vi "labviewRT_sm_example_waveform.vi"() -> ()   [LabVIEW 2019]
uses:
  lib/labviewRT-EPICS/linuxSharedMemory.lvlib
  lib/labviewRT-EPICS/sm u64 write and increment.vi
  lib/labviewRT-EPICS/sm single array write and increment.vi
  lib/labviewRT-EPICS/sm u64 write array and increment.vi
  lib/labviewRT-EPICS/sm u16 write array and increment.vi
  lib/labviewRT-EPICS/sm i64 write array and increment.vi
  lib/labviewRT-EPICS/sm double array write and increment.vi
  lib/labviewRT-EPICS/sm u32 write array and increment.vi
  lib/labviewRT-EPICS/sm i32 write and increment.vi
  lib/labviewRT-EPICS/sm u32 write and increment.vi
  lib/labviewRT-EPICS/sm u16 write and increment.vi
  lib/labviewRT-EPICS/sm i8 write and increment.vi
  lib/labviewRT-EPICS/sm bool write and increment.vi
  lib/labviewRT-EPICS/sm u8 write and increment.vi
  lib/labviewRT-EPICS/sm double write and increment.vi
  lib/labviewRT-EPICS/sm i8 write array and increment.vi
  lib/labviewRT-EPICS/sm i64 read and increment.vi
  lib/labviewRT-EPICS/sm i32 write array and increment.vi
  lib/labviewRT-EPICS/sm i16 write array and increment.vi
  lib/labviewRT-EPICS/sm bool array write and increment.vi
  lib/labviewRT-EPICS/sm u8 read and increment.vi
  lib/labviewRT-EPICS/sm u16 read and increment.vi
  lib/labviewRT-EPICS/sm i16 read and increment.vi
  lib/labviewRT-EPICS/sm u64 read and increment.vi
  lib/labviewRT-EPICS/sm i8 read and increment.vi
  lib/labviewRT-EPICS/sm single read and increment.vi
  lib/labviewRT-EPICS/sm i32 read and increment.vi
  lib/labviewRT-EPICS/sm single write and increment.vi
  lib/labviewRT-EPICS/sm u32 read and increment.vi
  lib/labviewRT-EPICS/sm i64 write and increment.vi
  lib/labviewRT-EPICS/sm u8 write array and increment.vi
  lib/labviewRT-EPICS/sm i16 write and increment.vi
  lib/labviewRT-EPICS/sm double read and increment.vi
  lib/labviewRT-EPICS/sm bool read and increment.vi
panel:
  in  "Boolean in scalar":bool
  in  "U8 scalar":u8
  in  "U16 scalar":u16
  in  "U32 scalar":u32
  in  "U64 scalar":u64
  in  "I8 scalar":i8
  in  "I16 scalar":i16
  in  "I32 scalar":i32
  in  "I64 scalar":i64
  in  "Sgl scalar":sgl format="%#_64g"
  in  "Dbl scalar":dbl format="%#_64g"
  out "U8 scalar":u8
  out "U16 scalar":u16
  out "U32 scalar":u32
  out "U64 scalar":u64
  out "I8 scalar":i8
  out "I16 scalar":i16
  out "I32 scalar":i32
  out "I64 scalar":i64
  out "Sgl  scalar":sgl format="%#_64g"
  out "Dbl scalar":dbl format="%#_64g"
  out "Boolean scalar":bool
  in  "stop":bool
  out "error out":errorcluster
  in  "u64 scaler":u64
  in  "i32":i32[](array[numeric])=[0, 0, 0, 0, 0, 0, 0, 0, 0, 1]
  in  "i16":i16[](array[numeric])=[0, 0, 0, 1]
  in  "i8":i8[](array[numeric])=[0, 0, 0, 0, 0, 0, 0, 1]
  in  "bool":bool[](array[boolean])=[FALSE, FALSE, FALSE, FALSE, FALSE, TRUE]
  in  "u64":u64[](array[numeric])=[0, 0, 0, 0, 0, 0, 0, 0, 1]
  in  "u16":u16[](array[numeric])=[0, 0, 0, 0, 0, 0, 0, 0, 0, 0, 1]
  in  "i64":i64[](array[numeric])=[0, 0, 0, 0, 1]
  in  "u8":u8[](array[numeric])=[0, 0, 0, 0, 0, 0, 0, 0, 1]
  out "Bool out":bool
  in  "double":dbl[](array[numeric])=[0.0, 0.0, 0.0, 1.0]
  in  "Shared Memory Size (bytes)":u32=4096
  in  "u32":u32[](array[numeric])=[0, 0, 0, 0, 0, 0, 0, 0, 0, 0, 0, 0, 0, 0, 0, 0, 0, 0, 0, 0, 0, 0, 0, 0, 0, 0, 0, 0, 0, 0, 0, 0, 0, 0, 0, 0, 0, 0, 0, 0, 0, 0, 0, 0, 0, 0, 0, 0, 0, 0, 0, 0, 0, 0, 0, 0, 0, 0, 0, 0, 0, 0, 0, 0, 0, 0, 0, 0, 0, 0, 0, 0, 0, 0, 0, 0, 0, 0, 0, 0, 0, 0, 0, 0, 0, 0, 0, 0, 0, 0, 0, 0, 0, 0, 0, 0, 0, 0, 0, 0, 0, 0, 0, 0, 0, 0, 0, 0, 0, 0, 0, 0, 1]
  in  "single":sgl[](array[numeric])=[0.0, 0.0, 0.0, 0.0, 1.0]
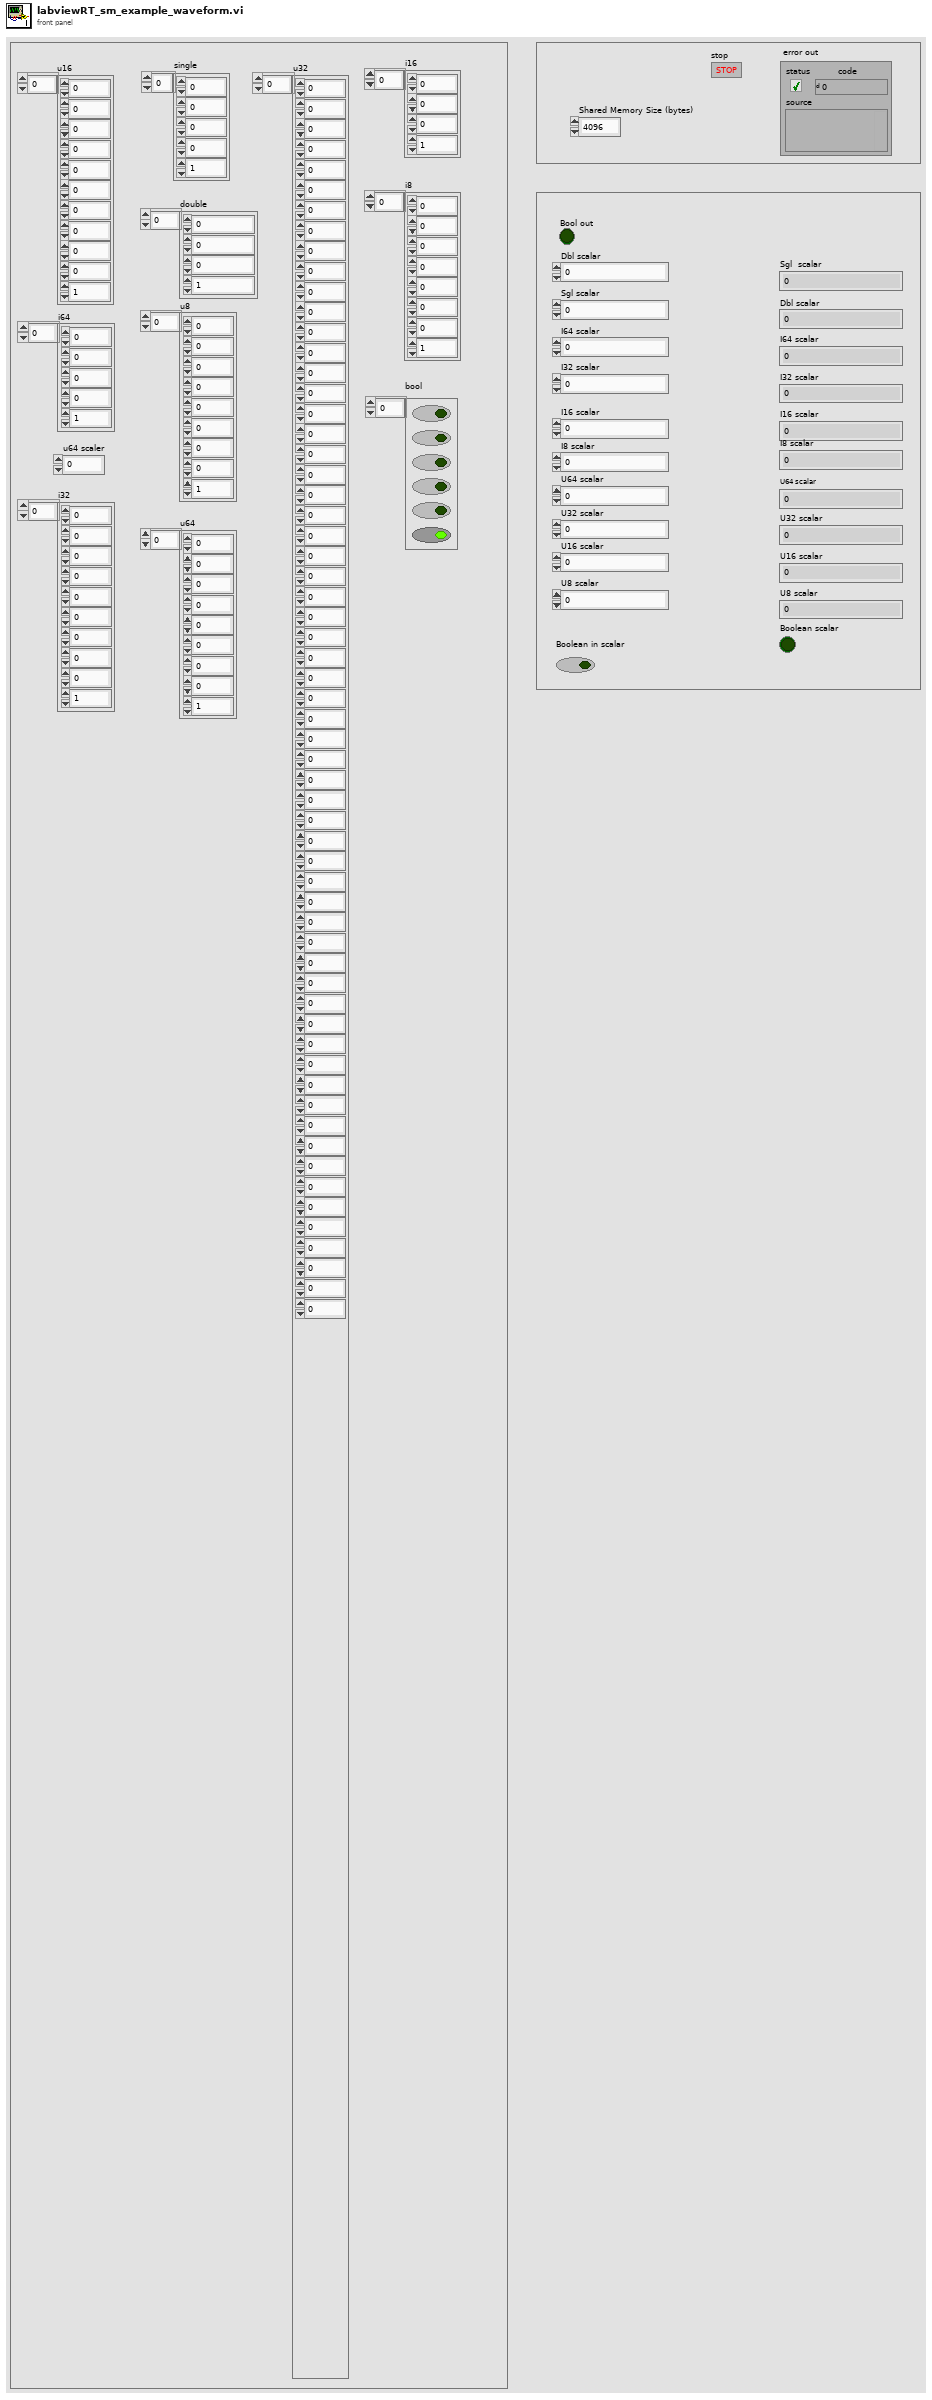
[diagram p1: front panel]
types:
  T1 = typedef "linuxSharedMemory.lvlib/sm_cluster.ctl" = cluster{"rt list":string, "error (no error)":errorcluster, "pointer":u64, "upper bound ptr":u64}
  T2 = typedef "Linux RT IPC.Shared Memory.lvlib/reference.ctl" = refnum<data-value>
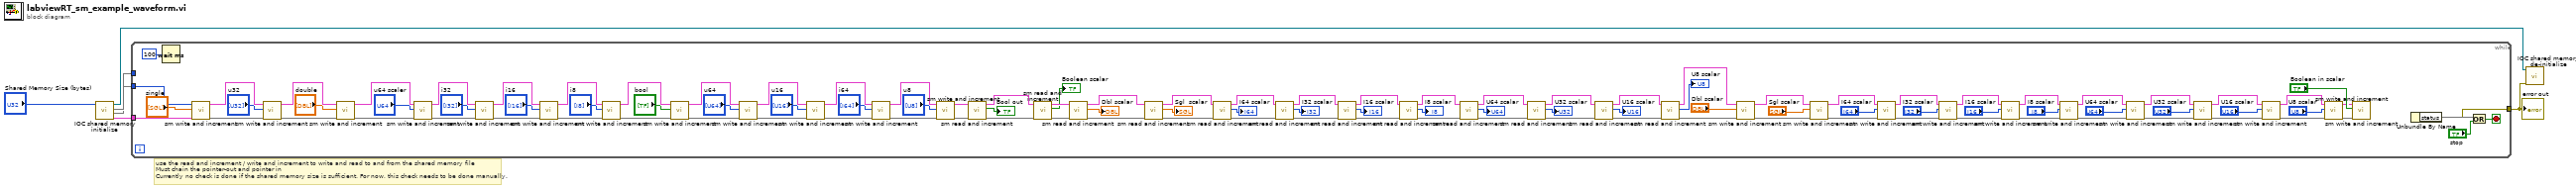
[diagram p0: block diagram]
diagram:
  # "use the read and increment / write and increment to write and read to and from the shared memory file\nMust chain the pointer-out and pointer in\nCurrently no check is done if the shared memory size is sufficient. For now, this check needs to be done manually."
  n1 = call "IOC shared memory initialize.vi"("Shared Memory Size (bytes)"="Shared Memory Size (bytes)") -> ("Shared memory cluster"=w5:T1, 1:w3, 2:w6, "shared memory class"=w1:T2)  [unwired: 7 in]
  n2 = while {
    tunnel: w6 -> [w118]
    tunnel: w5 -> [w116]
    tunnel: [w75] -> w2
    tunnel: w3 -> [w7]
    stop <- w76 stop-if-true
    n3 = Wait (ms)(milliseconds to wait=u32 100) -> ()  [unwired: 1 out]
    n4 = call-poly "sm write and increment.vi"(8:w116, "value in"="single", "Shared memory cluster"=w118) -> (0:w115, "Shared memory cluster output"=w114:T1)  [unwired: 7 in]
    n5 = call-poly "sm write and increment.vi"(8:w115, "value in"="u32", "Shared memory cluster"=w114) -> (0:w111, "Shared memory cluster output"=w110:T1)  [unwired: 7 in]
    n6 = call-poly "sm write and increment.vi"(8:w111, "value in"="double", "Shared memory cluster"=w110) -> (0:w99, "Shared memory cluster output"=w98:T1)  [unwired: 7 in]
    n7 = call-poly "sm write and increment.vi"(8:w99, "value in"="u64 scaler", "Shared memory cluster input"=w98) -> (0:w107, "Shared memory cluster output"=w97:T1)  [unwired: 7 in]
    n8 = call-poly "sm write and increment.vi"(8:w107, "value in"="i32", "Shared memory cluster"=w97) -> (0:w108, "Shared memory cluster output"=w96:T1)  [unwired: 7 in]
    n9 = call-poly "sm write and increment.vi"(8:w108, "value in"="i16", "Shared memory cluster"=w96) -> (0:w106, "Shared memory cluster output"=w95:T1)  [unwired: 7 in]
    n10 = call-poly "sm write and increment.vi"(8:w106, "value in"="i8", "Shared memory cluster"=w95) -> (0:w105, "Shared memory cluster output"=w94:T1)  [unwired: 7 in]
    n11 = call-poly "sm write and increment.vi"(8:w105, "value in"="bool", "Shared memory cluster"=w94) -> (0:w104, "Shared memory cluster output"=w93:T1)  [unwired: 7 in]
    n12 = call-poly "sm write and increment.vi"(8:w104, "value in"="u64", "Shared memory cluster"=w93) -> (0:w103, "Shared memory cluster output"=w92:T1)  [unwired: 7 in]
    n13 = call-poly "sm write and increment.vi"(8:w103, "value in"="u16", "Shared memory cluster"=w92) -> (0:w102, "Shared memory cluster output"=w91:T1)  [unwired: 7 in]
    n14 = call-poly "sm write and increment.vi"(8:w102, "value in"="i64", "Shared memory cluster"=w91) -> (0:w101, "Shared memory cluster output"=w90:T1)  [unwired: 7 in]
    n15 = call-poly "sm write and increment.vi"(8:w101, "value in"="u8", "Shared memory cluster"=w90) -> (0:w100, "Shared memory cluster output"=w89:T1)  [unwired: 7 in]
    n16 = call-poly "sm read and increment.vi"("Identifier"=w100, "Shared memory cluster input"=w89) -> (0:w11, "Bool out"=→"Bool out":bool, "Shared memory cluster output"=w9:T1)  [unwired: 7 in]
    n17 = call-poly "sm read and increment.vi"("Identifier"=w11, "Shared memory cluster input"=w9) -> (0:w13, "Bool out"=→"Boolean scalar":bool, "Shared memory cluster output"=w21:T1)  [unwired: 7 in]
    n18 = call-poly "sm read and increment.vi"("Identifier"=w13, "Shared memory cluster input"=w21) -> (0:w14, "Value out"=→"Dbl scalar":dbl, "Shared memory cluster output"=w22:T1)  [unwired: 7 in]
    n19 = call-poly "sm read and increment.vi"("Identifier"=w14, "Shared memory cluster input"=w22) -> (0:w15, "Value out"=→"Sgl  scalar":sgl, "Shared memory cluster output"=w23:T1)  [unwired: 7 in]
    n20 = call-poly "sm read and increment.vi"("Identifier"=w15, "Shared memory cluster input"=w23) -> (0:w16, "Value out"=→"I64 scalar":i64, "Shared memory cluster output"=w24:T1)  [unwired: 7 in]
    n21 = call-poly "sm read and increment.vi"("Identifier"=w16, "Shared memory cluster input"=w24) -> (0:w17, "Value out"=→"I32 scalar":i32, "Shared memory cluster output"=w25:T1)  [unwired: 7 in]
    n22 = call-poly "sm read and increment.vi"("Identifier"=w17, "Shared memory cluster input"=w25) -> (0:w18, "Value out"=→"I16 scalar":i16, "Shared memory cluster output"=w26:T1)  [unwired: 7 in]
    n23 = call-poly "sm read and increment.vi"("Identifier"=w18, "Shared memory cluster input"=w26) -> (0:w19, "Value out"=→"I8 scalar":i8, "Shared memory cluster output"=w27:T1)  [unwired: 7 in]
    n24 = call-poly "sm read and increment.vi"("Identifier"=w19, "Shared memory cluster input"=w27) -> (0:w20, "Value out"=→"U64 scalar":u64, "Shared memory cluster output"=w28:T1)  [unwired: 7 in]
    n25 = call-poly "sm read and increment.vi"("Identifier"=w20, "Shared memory cluster input"=w28) -> (0:w29, "Value out"=→"U32 scalar":u32, "Shared memory cluster output"=w32:T1)  [unwired: 7 in]
    n26 = call-poly "sm read and increment.vi"("Identifier"=w29, "Shared memory cluster input"=w32) -> (0:w31, "Value out"=→"U16 scalar":u16, "Shared memory cluster output"=w30:T1)  [unwired: 7 in]
    n27 = call-poly "sm read and increment.vi"("Identifier"=w31, "Shared memory cluster input"=w30) -> (0:w53, "Value out"=→"U8 scalar":u8, "Shared memory cluster output"=w8:T1)  [unwired: 7 in]
    n28 = call-poly "sm write and increment.vi"(8:w53, "value in"="Dbl scalar", "Shared memory cluster input"=w8) -> (0:w52, "Shared memory cluster output"=w55:T1)  [unwired: 7 in]
    n29 = call-poly "sm write and increment.vi"(8:w52, "value in"="Sgl scalar", "Shared memory cluster input"=w55) -> (0:w51, "Shared memory cluster output"=w56:T1)  [unwired: 7 in]
    n30 = call-poly "sm write and increment.vi"(8:w51, "value in"="I64 scalar", "Shared memory cluster input"=w56) -> (0:w50, "Shared memory cluster output"=w57:T1)  [unwired: 7 in]
    n31 = call-poly "sm write and increment.vi"(8:w50, "value in"="I32 scalar", "Shared memory cluster input"=w57) -> (0:w49, "Shared memory cluster output"=w58:T1)  [unwired: 7 in]
    n32 = call-poly "sm write and increment.vi"(8:w49, "value in"="I16 scalar", "Shared memory cluster input"=w58) -> (0:w48, "Shared memory cluster output"=w59:T1)  [unwired: 7 in]
    n33 = call-poly "sm write and increment.vi"(8:w48, "value in"="I8 scalar", "Shared memory cluster input"=w59) -> (0:w47, "Shared memory cluster output"=w60:T1)  [unwired: 7 in]
    n34 = call-poly "sm write and increment.vi"(8:w47, "value in"="U64 scalar", "Shared memory cluster input"=w60) -> (0:w46, "Shared memory cluster output"=w61:T1)  [unwired: 7 in]
    n35 = call-poly "sm write and increment.vi"(8:w46, "value in"="U32 scalar", "Shared memory cluster input"=w61) -> (0:w45, "Shared memory cluster output"=w62:T1)  [unwired: 7 in]
    n36 = call-poly "sm write and increment.vi"(8:w45, "value in"="U16 scalar", "Shared memory cluster input"=w62) -> (0:w44, "Shared memory cluster output"=w63:T1)  [unwired: 7 in]
    n37 = call-poly "sm write and increment.vi"(8:w44, "value in"="U8 scalar", "Shared memory cluster input"=w63) -> (0:w43, "Shared memory cluster output"=w64:T1)  [unwired: 7 in]
    n38 = call-poly "sm write and increment.vi"(8:w43, "value in"="Boolean in scalar", "Shared memory cluster input"=w64) -> (0:w10)  [unwired: 7 in, 1 out]
    n39 = Unbundle By Name() -> (w75:errorcluster, "status"=w77)
    n40 = Or(x=w77, y="stop") -> (x .or. y?=w76:bool)
  }
  "error out" <- w2
  n41 = call "IOC shared memory de-initialize.vi"("shared memory in"=w1, "Shared memory cluster"=w2) -> ()  [unwired: 9 in]
